vi "Connection Monitor.vi"(7 "Continuous Tasks Polling Rate in":i32, 8 "error in":errorcluster, 10 "Module ID":i32=-1, 11 "VISA Refnum in":refnum<visa-resource-name>) -> (0 "error out":errorcluster, 3 "VISA Refnum out":refnum<visa-resource-name>, 5 "Continuous Tasks Polling Rate out":i32)   [LabVIEW 2024, in "CTIWrapper.lvlib"]
uses:
  CTIWrapper.lvlib
  52334daa-c06b-4ced-9255-e18923a6b4a0.vi
  <instrlib>/HandsOnPi2040/HandsOnPi2040.lvlib
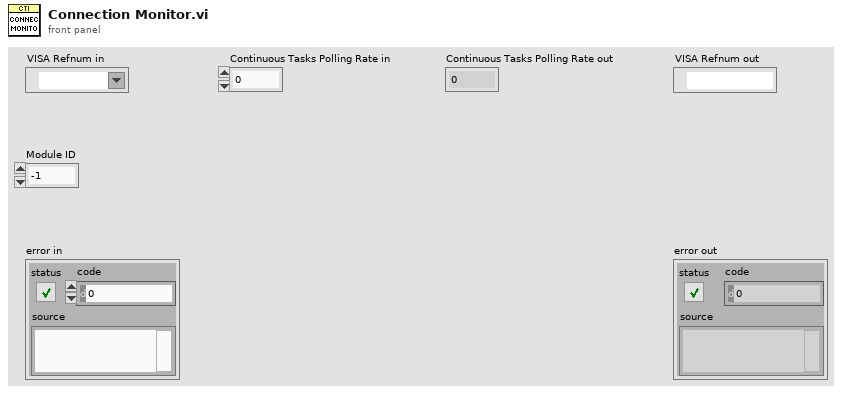
[diagram p1: front panel]
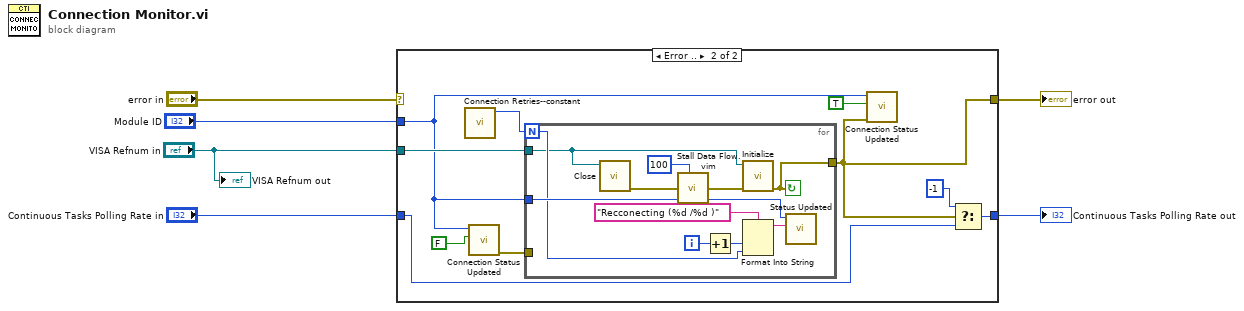
[diagram p0: block diagram]
diagram:
  n1 = case shown="Error .." "error in" {
    selector: "error in" -> [w8 _]
    tunnel: [w8 w17] -> w5
    tunnel: "Continuous Tasks Polling Rate in" -> [w7 w14]
    tunnel: [w7 w13] -> w3
    tunnel: "VISA Refnum in" -> [_ w16]
    tunnel: "Module ID" -> [_ w9]
    frame No Error {
      # "No Error do Nothing"
    }
    frame Error {
      n2 = call "Connection Retries--constant.vi"() -> ("Retries"=w11:i32)  [unwired: 11 in]
      n3 = call "Connection Status Updated.vi"("Connected?"=FALSE, "Module ID"=w9) -> ("error out"=w18:errorcluster)  [unwired: 9 in]
      n4 = for {
        N: w11 -> [w20]
        tunnel: w16 -> [w19]
        tunnel: w18 -> [_]
        tunnel: [w28] -> w17
        tunnel: w9 -> [w25]
        i -> [w23]
        stop <- w28 continue-if-true
        n5 = call <instrlib>:"Close.vi"("VISA resource name"=w19) -> ("error out"=w29:errorcluster)  [unwired: 10 in]
        n6 = call "Stall Data Flow.vim"("value in"=w29, "milliseconds to wait"=u32 100) -> ("value out"=w27:errorcluster)  [unwired: 1 out]
        n7 = Increment(x=w23) -> (x+1=w22:i32)
        n8 = call <instrlib>:"Initialize.vi"("error in (no error)"=w27, "VISA resource name"=w19) -> ("error out"=w28:errorcluster)  [unwired: 7 in, 2 out]
        n9 = Format Into String(format string="Recconecting (%d /%d )", w22, w20) -> (resulting string=w24:string)  [unwired: 2 in, 1 out]
        n10 = call "Status Updated.vi"("Status"=w24, "Module ID"=w25) -> ()  [unwired: 9 in, 1 out]
      }
      n11 = call "Connection Status Updated.vi"("error in"=w17, "Connected?"=TRUE, "Module ID"=w9) -> ()  [unwired: 8 in, 1 out]
      n12 = Select(t=-1, s=w17, f=w14) -> (s? t:f=w13:i32)
    }
  }
  "error out" <- w5
  "Continuous Tasks Polling Rate out" <- w3
  "VISA Refnum out" <- "VISA Refnum in"
